vi "Trav_pos_for_Email.vi"() -> (0 "String":string)   [LabVIEW 2015]
uses:
  Controls/Overhead.ctl
  Globals/Trav_pos_global.vi
  Globals/Meas_global.vi
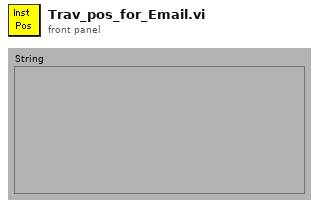
[diagram p1: front panel]
types:
  T1 = typedef "Overhead.ctl" = enum16{"Update total times", "Read Current Overhead", "Re Scale totals to 3 hrs", "Initialise totals to 3hr"}
  T2 = typedef "Tunnel_Coordinates.ctl" = enum16{"Work in Tunnel Coordinates", "Work in Model Coordinates"}
  T3 = typedef "Traverse_cluster.ctl" = cluster{"Start X":sgl, "Start Y":sgl, "Start Z":sgl, "End X":sgl, "End Y":sgl, "End Z":sgl, "No. of pts.":i32, "Spacing":T4, "Filename":path, "Tunnel Speed":dbl, "Averaging time (min)":dbl, "Extra Commands":string, "Carrier_1 Q (l/min)":dbl, "Carrier_2 Q (l/min)":dbl, "Trace Gas Concentration (%)":dbl, "Specific Arguments":string, "Comments":string, "Row No":i32, "Row Type Selector":T5, "Completion time":string, "Row Duration (mins)":dbl, "No. of Valid pts.":i32, "Meas Setup File":string}
  T4 = typedef "Spacing.ctl" = enum16{"Linear", "Log", "Gauss", "Specified", "N/A"}
  T5 = typedef "Multi_run_mode.ctl" = enum16{"Move Traverse Only", "Set Tunnel Speed Only", "Set Source Only", "Set Measurement Conditions", "Single Measurement", "Vertical Profile", "Lateral Profile", "Longitudinal Profile", "Explore Volume", "Multi-Axis Profile", "Auto Calibrate", "Meas Fast FID Bkgnd", "Check Beam Power", "Scanning Valve Measurement", "Run VI Named:", "Set ADAM Ch", "Wait (minutes)", "Send Message", "Synchronize With:", "Fall Back to this Row", "Turn Off Row Repeating", "Blank Row", "Traverse 3D Volume"}
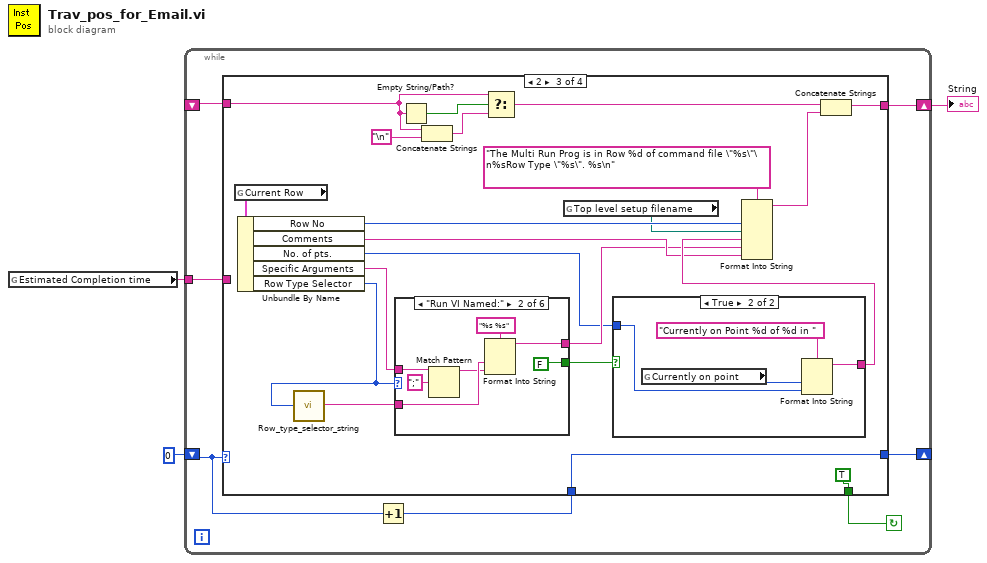
[diagram p0: block diagram]
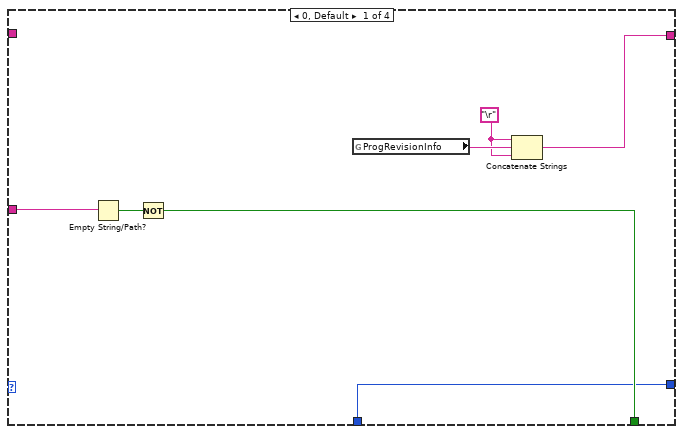
[diagram p2: hidden frame]
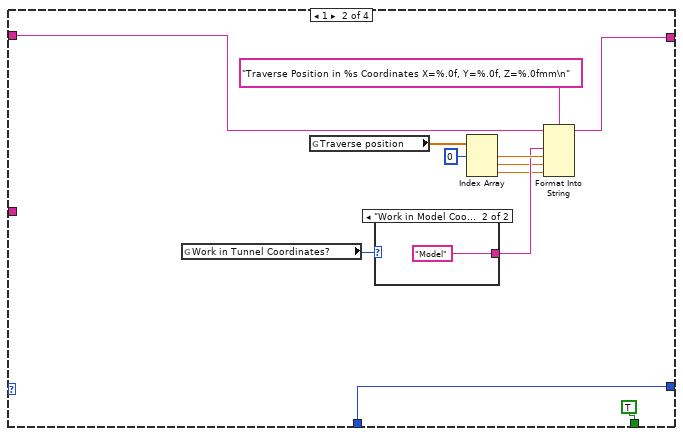
[diagram p3: hidden frame]
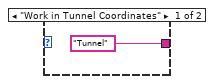
[diagram p4: hidden frame]
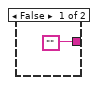
[diagram p5: hidden frame]
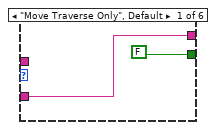
[diagram p6: hidden frame]
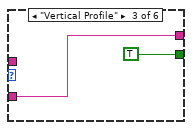
[diagram p7: hidden frame]
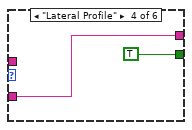
[diagram p8: hidden frame]
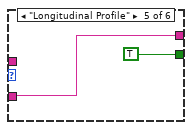
[diagram p9: hidden frame]
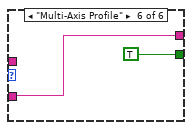
[diagram p10: hidden frame]
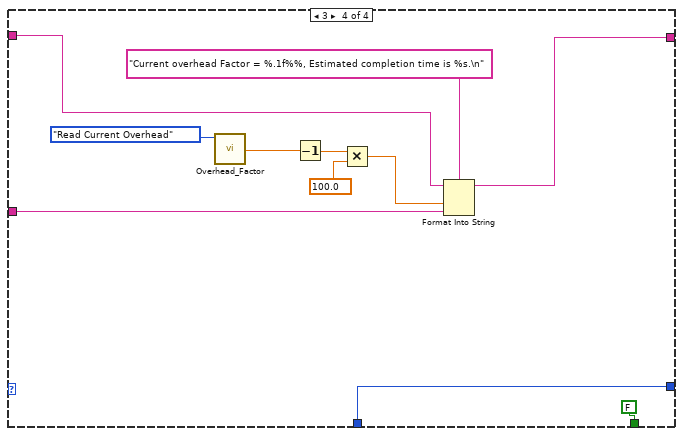
[diagram p11: hidden frame]
diagram:
  n1 = global read "Trav_pos_global.vi" "Estimated Completion time"() -> (w1:string)
  n2 = while {
    shift-left: _ -> [w5]
    shift-right: [w7] -> w2
    shift-left: 0 -> [w10]
    shift-right: [w9] -> _
    tunnel: w1 -> [w4]
    stop <- w6 continue-if-true
    n3 = Increment(x=w10) -> (x+1=w8:i32)
    n4 = case shown="2" w10 {
      tunnel: [w14 w29 w47 w84] -> w9
      tunnel: w8 -> [w14 w29 w47 w84]
      tunnel: [w12 w24 w52 w76] -> w7
      tunnel: [w15 TRUE TRUE FALSE] -> w6
      tunnel: w5 -> [_ w25 w44 w77]
      tunnel: w4 -> [w17 _ _ w75]
      frame 0, Default {
        w11 = "\r"
        n5 = Empty String/Path?(string/path=w17) -> (empty?=w16:bool)
        n6 = Not(x=w16) -> (.not. x?=w15:bool)
        n7 = global read "Meas_global.vi" "ProgRevisionInfo"() -> (w13:string)
        n8 = Concatenate Strings(w11, w13, w11) -> (w12:string)
      }
      frame 1 {
        n9 = global read "Trav_pos_global.vi" "Work in Tunnel Coordinates?"() -> (w23:T2)
        n10 = global read "Trav_pos_global.vi" "Traverse position"() -> (w20:sgl[])
        n11 = case shown="\"Work in Model Coordinates\"" w23 {
          tunnel: ["Tunnel" "Model"] -> w21
          frame "Work in Tunnel Coordinates" {
          }
          frame "Work in Model Coordinates" {
          }
        }
        n12 = Index Array(array=w20, index #1=0 ("index")) -> (element #1=w22:sgl, element #2=w19:sgl, element #3=w18:sgl)  [unwired: 2 in]
        n13 = Format Into String(format string="Traverse Position in %s Coordinates X=%.0f, Y=%.0f, Z=%.0fmm\n" ("Format String"), initial string=w25, w21, w22, w19, w18) -> (resulting string=w24:string)  [unwired: 1 in, 1 out]
      }
      frame 2 {
        n14 = global read "Trav_pos_global.vi" "Current Row"() -> (w38:T3)
        n15 = Unbundle By Name(w38) -> ("Row No"=w51:i32, "Comments"=w37:string, "No. of pts."=w32:i32, "Specific Arguments"=w34:string, "Row Type Selector"=w33:T5)
        n16 = call "Row_type_selector_string.vi"("Mode"=w33) -> ("Output string"=w36:string)
        n17 = case shown="\"Run VI Named:\"" w33 {
          tunnel: [FALSE FALSE TRUE TRUE TRUE TRUE] -> w50
          tunnel: w36 -> [w58 w65 w67 w69 w71 w73]
          tunnel: [w58 w63 w67 w69 w71 w73] -> w35
          tunnel: w34 -> [_ w61 _ _ _ _]
          frame "Move Traverse Only", Default {
          }
          frame "Run VI Named:" {
            n18 = Match Pattern(string=w61, regular expression=";") -> (before substring=w60:string)  [unwired: 4 out]
            n19 = Format Into String(format string="%s %s" ("Format String"), w65, w60) -> (resulting string=w63:string)  [unwired: 2 in, 1 out]
          }
          frame "Vertical Profile" {
          }
          frame "Lateral Profile" {
          }
          frame "Longitudinal Profile" {
          }
          frame "Multi-Axis Profile" {
          }
        }
        n20 = Empty String/Path?(string/path=w44) -> (empty?=w46:bool)
        n21 = Concatenate Strings(w44, "\n") -> (w45:string)
        n22 = Select(t=w44, s=w46, f=w45) -> (s? t:f=w43:string)
        n23 = global read "Trav_pos_global.vi" "Top level setup filename"() -> (w41:path)
        n24 = case shown="True" w50 {
          tunnel: w32 -> [_ w56]
          tunnel: ["" w54] -> w40
          frame False {
          }
          frame True {
            n25 = global read "Trav_pos_global.vi" "Currently on point"() -> (w57:i32)
            n26 = Format Into String(format string="Currently on Point %d of %d in " ("Format String"), w57, w56) -> (resulting string=w54:string)  [unwired: 2 in, 1 out]
          }
        }
        n27 = Format Into String(format string="The Multi Run Prog is in Row %d of command file \"%s\"\n%sRow Type \"%s\". %s\n" ("Format String"), w51, w41, w40, w35, w37) -> (resulting string=w39:string)  [unwired: 2 in, 1 out]
        n28 = Concatenate Strings(w43, w39) -> (w52:string)
      }
      frame 3 {
        n29 = call "Overhead_Factor.vi"("Mode"=Overhead."Read Current Overhead") -> ("Current Overhead Factor"=w82:dbl)  [unwired: 3 in]
        n30 = Decrement(x=w82) -> (x-1=w81:dbl)
        n31 = Multiply(x=w81, y=100.0) -> (x*y=w79:dbl)
        n32 = Format Into String(format string="Current overhead Factor = %.1f%%, Estimated completion time is %s.\n" ("Format String"), initial string=w77, w79, w75) -> (resulting string=w76:string)  [unwired: 1 in, 1 out]
      }
    }
  }
  "String" <- w2
